vi "interface_select_project.vi"(8 "error in (no error)":errorcluster) -> (0 "error out":errorcluster, 3 "project_path":path)   [LabVIEW 2015, in "lv-build-interface.lvlib"]
uses:
  lv-build-interface.lvlib
  <vilib>/Utility/error.llb/Error Cluster From Error Code.vi
  <vilib>/ErrorRing/Error Ring.xnode
panel:
  in  "refresh":bool
  in  "select_project":bool
  in  "tree":i32(listbox)
  in  "open_project":bool
  in  "cancel":bool
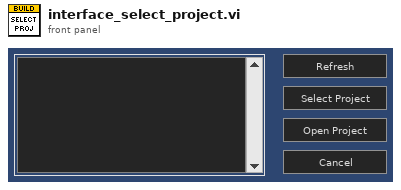
[diagram p1: front panel]
types:
  T1 = enum8{"Enabled", "Disabled", "Disabled and Grayed Out"}
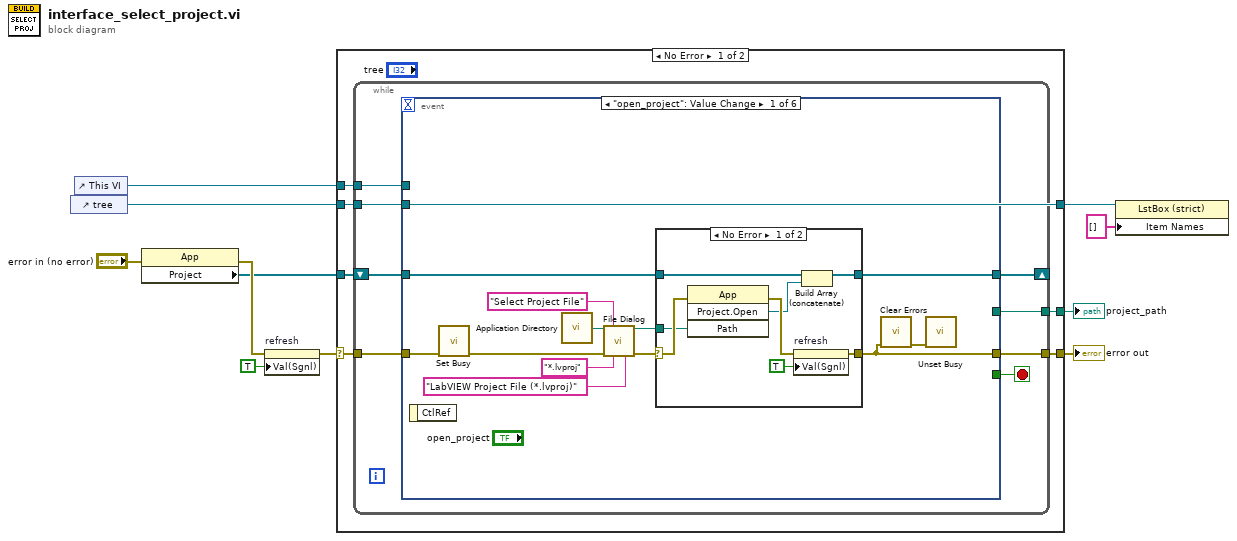
[diagram p0: block diagram]
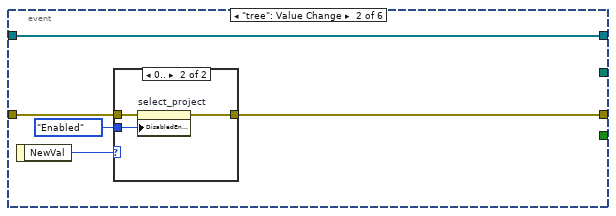
[diagram p3: hidden frame]
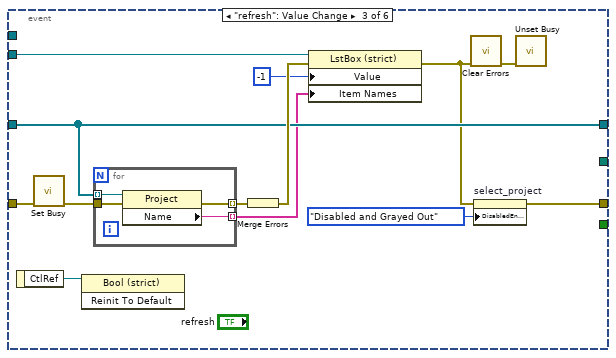
[diagram p5: hidden frame]
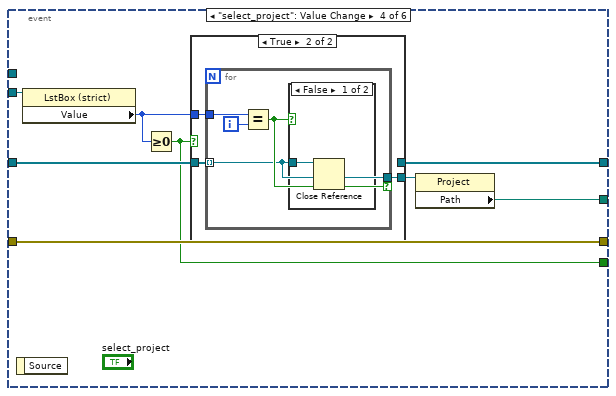
[diagram p6: hidden frame]
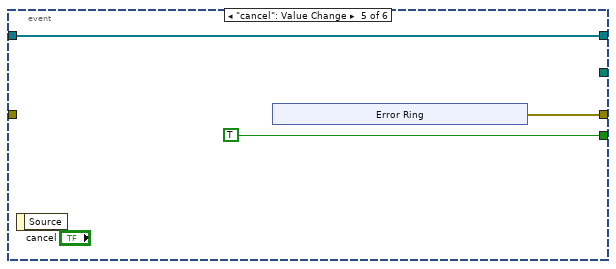
[diagram p9: hidden frame]
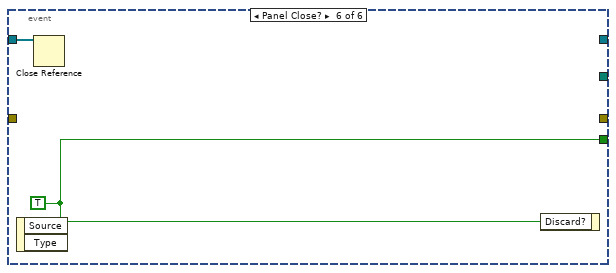
[diagram p10: hidden frame]
diagram:
  n1 = control-ref of="tree"() -> (w7:refnum<vi>)
  n2 = control-ref of="This VI"() -> (w4:refnum<vi>)
  n3 = property class="App"(error in="error in (no error)") -> (error out=w9:errorcluster, "Project"=w8:refnum<vi>[])  [unwired: 1 in, 1 out]
  n4 = property on="refresh" class="Bool (strict)"(error in=w9, "Val(Sgnl)"=TRUE ("Value (Signaling)")) -> (error out=w11:errorcluster)  [unwired: 1 in, 1 out]
  n5 = case shown="No Error" w11 {
    selector: w11 -> [w15 w101]
    tunnel: [w17 w101] -> w1
    tunnel: w4 -> [w16 _]
    tunnel: w7 -> [w12 w100]
    tunnel: w8 -> [w14 _]
    tunnel: [w13 _] -> w3
    tunnel: [w12 w100] -> w6
    frame No Error {
      n6 = while {
        tunnel: [w25] -> w17
        tunnel: w15 -> [w24]
        tunnel: w16 -> [w18]
        tunnel: w12 -> [w23]
        shift-right: [w20] -> _
        shift-left: w14 -> [w21]
        tunnel: [w19] -> w13
        stop <- w22 stop-if-true
        n7 = event shown="[0] \"open_project\": Value Change" {
          selector: _ -> [_ _ _ _ _ _]
          dyn-events: _ -> [_ _ _ _ _ _]
          timeout: _ -> [_ _ _ _ _ _]
          tunnel: [w33 w48 w58 w80 w91 _] -> w25
          tunnel: w24 -> [w35 w49 w61 w80 _ _]
          tunnel: w18 -> [_ _ _ _ _ _]
          tunnel: w23 -> [_ _ w66 w81 _ _]
          tunnel: [_ _ _ w76 TRUE w99] -> w22
          tunnel: w21 -> [w37 w52 w65 w78 w92 w98]
          tunnel: [w36 w52 w65 w77 w92 _] -> w20
          tunnel: [_ _ _ w74 _ _] -> w19
          event "open_project": Value Change {
            n8 = event-data() -> ()  [unwired: 1 in, 1 out]
            n9 = call <vilib>:"Set Busy.vi"("error in (no error)"=w35) -> ("error out"=w32:errorcluster)  [unwired: 9 in, 1 out]
            n10 = call <vilib>:"Application Directory.vi"() -> ("Application Directory"=w29:path)
            n11 = call "File Dialog"("start path"=w29, "prompt"="Select Project File", "error in"=w32, "pattern (all files)"="*.lvproj" ("filter"), "pattern label"="LabVIEW Project File (*.lvproj)" ("filter")) -> ("selected path"=w28:path, "error out"=w31:errorcluster)  [unwired: 7 in, 2 out]
            n12 = case shown="No Error" w31 {
              selector: w31 -> [w44 w47]
              tunnel: w28 -> [w43 _]
              tunnel: [w41 w47] -> w33
              tunnel: w37 -> [w39 w46]
              tunnel: [w38 w46] -> w36
              frame No Error {
                n13 = invoke class="App" method="Project.Open"(error in=w44, "Path"=w43) -> (error out=w42:errorcluster, "Project:Open"=w40:refnum<vi>)  [unwired: 2 in, 2 out]
                n14 = property on="refresh" class="Bool (strict)"(error in=w42, "Val(Sgnl)"=TRUE ("Value (Signaling)")) -> (error out=w41:errorcluster)  [unwired: 1 in, 1 out]
                n15 = Build Array (concatenate)(w39, w40) -> (w38:refnum<vi>[])
              }
              frame Error {
              }
            }
            n16 = call <vilib>:"Clear Errors.vi"("error in (no error)"=w33) -> ("error out"=w34:errorcluster)  [unwired: 5 in, 1 out]
            n17 = call <vilib>:"Unset Busy.vi"("error in (no error)"=w34) -> ()  [unwired: 10 in, 1 out]
          }
          event "tree": Value Change {
            n18 = event-data() -> ("NewVal"=w50:i32)  [unwired: 1 in]
            n19 = case shown="0.." w50 {
              tunnel: T1."Enabled" ("Disabled") -> [_ w56]
              tunnel: w49 -> [w53 w55]
              tunnel: [w53 w54] -> w48
              frame Default {
              }
              frame 0.. {
                n20 = property on="select_project" class="Bool"(error in=w55, "DisabledEnum"=w56) -> (error out=w54:errorcluster)  [unwired: 1 in, 1 out]
              }
            }
          }
          event "refresh": Value Change {
            n21 = event-data() -> ("CtlRef"=w67:refnum<vi>)  [unwired: 1 in]
            n22 = call <vilib>:"Set Busy.vi"("error in (no error)"=w61) -> ("error out"=w60:errorcluster)  [unwired: 9 in, 1 out]
            n23 = invoke class="Bool (strict)" method="Reinit To Default"(reference=w67) -> ()  [unwired: 2 in, 3 out]
            n24 = for {
              tunnel: [w73] -> w63 mode=indexing
              tunnel: w65 -> [w72] mode=indexing
              tunnel: w60 -> [w71]
              tunnel: [w70] -> w68 mode=indexing
              n25 = property class="Project"(reference=w72, error in=w71) -> (error out=w70:errorcluster, "Name"=w73:string)  [unwired: 1 out]
            }
            n26 = Merge Errors(w68) -> (w69:errorcluster)
            n27 = property class="LstBox (strict)"(reference=w66, error in=w69, "Value"=-1, "Item Names"=w63) -> (error out=w59:errorcluster)  [unwired: 1 out]
            n28 = call <vilib>:"Clear Errors.vi"("error in (no error)"=w59) -> ("error out"=w62:errorcluster)  [unwired: 5 in, 1 out]
            n29 = property on="select_project" class="Bool"(error in=w59, "DisabledEnum"=T1."Disabled and Grayed Out" ("Disabled")) -> (error out=w58:errorcluster)  [unwired: 1 in, 1 out]
            n30 = call <vilib>:"Unset Busy.vi"("error in (no error)"=w62) -> ()  [unwired: 10 in, 1 out]
          }
          event "select_project": Value Change {
            n31 = event-data() -> ()  [unwired: 1 in, 1 out]
            n32 = property class="LstBox (strict)"(reference=w81) -> ("Value"=w79:i32)  [unwired: 1 in, 2 out]
            n33 = Greater Or Equal To 0?(x=w79) -> (x >= 0?=w76:bool)
            n34 = case shown="True" w76 {
              tunnel: [_ w85] -> w75
              tunnel: w79 -> [_ w84]
              tunnel: w78 -> [w82 w83]
              tunnel: [w82 _] -> w77
              frame False {
              }
              frame True {
                n35 = for {
                  tunnel: w83 -> [w86] mode=indexing
                  tunnel: w84 -> [w89]
                  tunnel: [w86] -> w85 if=w87
                  i -> [w88]
                  n36 = Equal?(x=w89, y=w88) -> (x = y?=w87:bool)
                  n37 = case shown="False" w87 {
                    tunnel: w86 -> [w90 _]
                    frame False {
                      n38 = Close Reference(reference=w90) -> ()  [unwired: 1 in, 1 out]
                    }
                    frame True {
                    }
                  }
                }
              }
            }
            n39 = property class="Project"(reference=w75) -> ("Path"=w74:path)  [unwired: 1 in, 2 out]
          }
          event "cancel": Value Change {
            n40 = event-data() -> ()  [unwired: 1 in, 1 out]
            n41 = xnode "Error Ring"() -> ("error out"=w91:errorcluster)
          }
          event Panel Close? {
            w99 = TRUE
            n42 = event-data() -> ()  [unwired: 1 in, 2 out]
            n43 = Close Reference(reference=w98) -> ()  [unwired: 1 in, 1 out]
            n44 = event-data("Discard?"=w99) -> ()  [unwired: 1 in, 1 out]
          }
        }
      }
    }
    frame Error {
    }
  }
  "project_path" <- w3
  "error out" <- w1
  n45 = property class="LstBox (strict)"(reference=w6, "Item Names"=string[] []) -> ()  [unwired: 1 in, 2 out]
